vi "ProcessBufferUpdates.vi"(11 "MockAccelSettings":T1={"BufferUpdateFIFO"="MockAccelVoltageFIFO"}) -> ()   [LabVIEW 2016, in "FPGAMockAccel.lvlib"]
uses:
  FPGAMockAccel.lvlib
  DataTypes/MockAccelSettings.ctl
  <vilib>/rvi/Emulation/niFpgaGetClockAttributes.vi
  <vilib>/rvi/Emulation/niFpgaSctlEmulationGetInTimedLoop.vi
  <vilib>/rvi/Emulation/niFpgaEmulationReportErrorSimple.vi
  <vilib>/rvi/DataTransferAndStorage/Container/Common/niFpgaContainerExecOnDevCompGetState.vi
  <vilib>/rvi/Emulation/niFpgaEmulationIsFPGAContextNoSignature.vi
  <vilib>/rvi/errors/niFpgaSetErrorForExecOnDevCompSimple.vi
  <vilib>/rvi/eio/common/nirviEmuReportErrorAndStop.vi
  <vilib>/rvi/DataTransferAndStorage/Container/Common/niFpgaContainerGetUniqueNameForEmu.vi
  <vilib>/rvi/FIFO/Fifo_Resource/nirvififoEmulationSetSize.vi
  <vilib>/rvi/FIFO/Fifo_Resource/nirviFifoEmulationQueueMgr.vi
  <instcachedir>/0/nirviFifoEmulationQueueMgr_E5CAEC123FF24DC58D834DCA3CDAA9B5.lvgen/nirviFifoEmulationQueueMgr_E5CAEC123FF24DC58D834DCA3CDAA9B5_009.vi
  <vilib>/rvi/FIFO/Fifo_Resource/nirvififoEmulationDetermineInputValidOut.vi
  <vilib>/rvi/FIFO/Fifo_Resource/nirvififoEmulationCreateLock.vi
  <vilib>/rvi/Emulation/niFpgaProcessEmulError.vi
  <vilib>/rvi/FIFO/Fifo_Resource/nirvififoEmulationObtainLock.vi
  <vilib>/rvi/FIFO/Fifo_Resource/nirvififoEmulationReleaseLock.vi
  <vilib>/rvi/occurrence/nirviWaitOnOccurrenceBase.vi
  <vilib>/rvi/errors/nirviReportUnexpectedCaseInternalError.vi
  <vilib>/rvi/errors/nirviReportUnexpectedCaseInternalError (U32).vi
  <vilib>/Utility/error.llb/Clear Errors.vi
  <vilib>/rvi/interface/RandomDataEmulation/niFpgaRandomDataHandleErrors.vi
  <vilib>/rvi/eio/common/nirviEmuTemplateMethod_errors.vi
  <vilib>/rvi/Emulation/niFpgaCriticalErrorInLSC.vi
  <vilib>/rvi/DataTransferAndStorage/Container/XNode/niFpgaContainer.xnode
  <vilib>/rvi/FIFO/Fifo_Resource/niFpgaFifoEmulationRefIn.vi
  <vilib>/eio/EIONode/EIONode.xnode
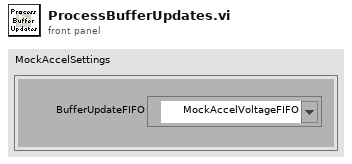
[diagram p1: front panel]
types:
  T1 = typedef "FPGAMockAccel.lvlib/MockAccelSettings.ctl" = cluster{"BufferUpdateFIFO":refnum<k21>}
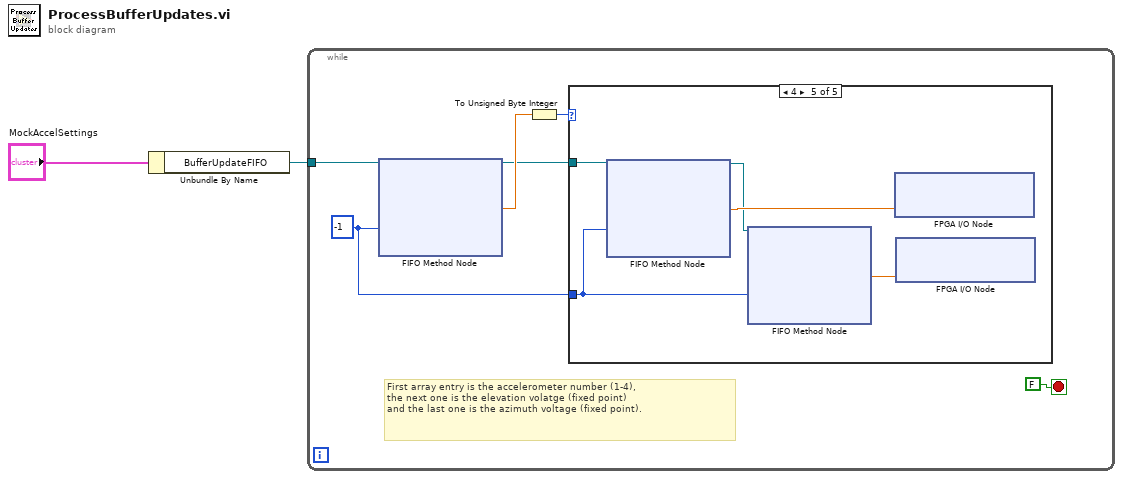
[diagram p0: block diagram]
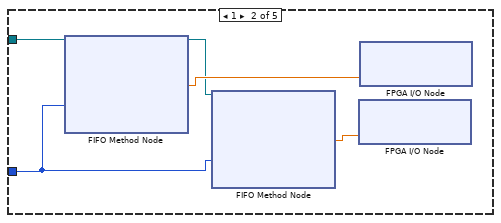
[diagram p3: hidden frame]
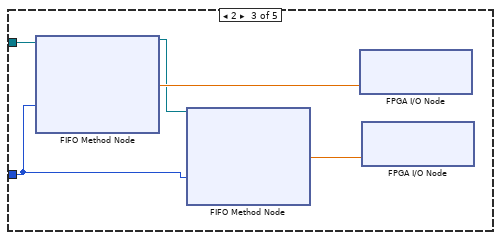
[diagram p4: hidden frame]
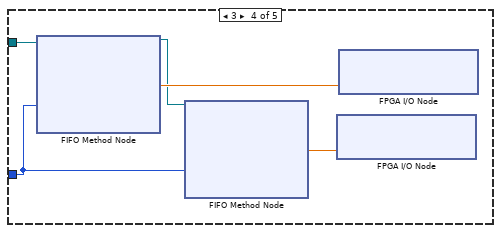
[diagram p5: hidden frame]
diagram:
  n1 = Unbundle By Name("MockAccelSettings") -> ("BufferUpdateFIFO"=w2:refnum<k21>)
  n2 = while {
    tunnel: w2 -> [w7]
    stop <- FALSE stop-if-true
    w4 = -1 ("Timeout")
    # "First array entry is the accelerometer number (1-4), \nthe next one is the elevation volatge (fixed point)\nand the last one is the azimuth voltage (fixed point)."
    n3 = xnode ("FIFO Method Node")("Timeout"=w4, "FIFO In"=w7) -> ("Element"=w6:sgl, "FIFO Out"=w3:refnum<k21>)  [unwired: 1 out]
    n4 = To Unsigned Byte Integer(number=w6) -> (unsigned 8bit integer=w5:u8)
    n5 = case shown="4" w5 {
      tunnel: w3 -> [_ w13 w18 w23 w28]
      tunnel: w4 -> [_ w10 w15 w19 w25]
      frame 0, Default {
      }
      frame 1 {
        n6 = xnode ("FIFO Method Node")("Timeout"=w10, "FIFO In"=w13) -> ("Element"=w12:sgl, "FIFO Out"=w11:refnum<k21>)  [unwired: 1 out]
        n7 = xnode ("FIFO Method Node")("Timeout"=w10, "FIFO In"=w11) -> ("Element"=w9:sgl)  [unwired: 2 out]
        n8 = xnode "FPGA I/O Node"("Slot1/AO1"=w9) -> ()  [unwired: 1 in, 1 out]
        n9 = xnode "FPGA I/O Node"("Slot1/AO0"=w12) -> ()  [unwired: 1 in, 1 out]
      }
      frame 2 {
        n10 = xnode ("FIFO Method Node")("Timeout"=w15, "FIFO In"=w18) -> ("Element"=w17:sgl, "FIFO Out"=w16:refnum<k21>)  [unwired: 1 out]
        n11 = xnode ("FIFO Method Node")("Timeout"=w15, "FIFO In"=w16) -> ("Element"=w14:sgl)  [unwired: 2 out]
        n12 = xnode "FPGA I/O Node"("Slot1/AO2"=w17) -> ()  [unwired: 1 in, 1 out]
        n13 = xnode "FPGA I/O Node"("Slot1/AO3"=w14) -> ()  [unwired: 1 in, 1 out]
      }
      frame 3 {
        n14 = xnode ("FIFO Method Node")("Timeout"=w19, "FIFO In"=w23) -> ("Element"=w22:sgl, "FIFO Out"=w21:refnum<k21>)  [unwired: 1 out]
        n15 = xnode ("FIFO Method Node")("Timeout"=w19, "FIFO In"=w21) -> ("Element"=w20:sgl)  [unwired: 2 out]
        n16 = xnode "FPGA I/O Node"("Slot2-AO/AO1"=w20) -> ()  [unwired: 1 in, 1 out]
        n17 = xnode "FPGA I/O Node"("Slot2-AO/AO0"=w22) -> ()  [unwired: 1 in, 1 out]
      }
      frame 4 {
        n18 = xnode ("FIFO Method Node")("Timeout"=w25, "FIFO In"=w28) -> ("Element"=w27:sgl, "FIFO Out"=w26:refnum<k21>)  [unwired: 1 out]
        n19 = xnode ("FIFO Method Node")("Timeout"=w25, "FIFO In"=w26) -> ("Element"=w24:sgl)  [unwired: 2 out]
        n20 = xnode "FPGA I/O Node"("Slot2-AO/AO2"=w27) -> ()  [unwired: 1 in, 1 out]
        n21 = xnode "FPGA I/O Node"("Slot2-AO/AO3"=w24) -> ()  [unwired: 1 in, 1 out]
      }
    }
  }
